vi "test_Local Chassis Number of Slots Property.vi"(8 "error in (no error)":errorcluster, 11 "TestCase in":refnum<class "Scan Engine Scripting API Custom Device Unit Tests.lvclass">) -> (0 "error out":errorcluster, 3 "TestCase out":refnum<class "Scan Engine Scripting API Custom Device Unit Tests.lvclass">)   [LabVIEW 2020, in "Scan Engine Scripting API Custom Device Unit Tests.lvclass"]
uses:
  Scan Engine Scripting API Custom Device Unit Tests.lvclass
  Shared/Type Defs/Main Settings.ctl
  Shared/Type Defs/Local Chassis Settings.ctl
  Scan Engine Scripting API Custom Device Unit Tests.lvclass/Scan Engine Scripting API Custom Device Unit Tests.ctl
  <vilib>/addons/_JKI Toolkits/VI Tester/TestCase.llb/TestCase.lvclass
  Scripting/Scan Engine Scripting.lvlib
  Shared/SEECD Shared.lvlib
  C:/Program Files (x86)/National Instruments/LabVIEW 2020/vi.lib/addons/_JKI Toolkits/VI Tester/TestCase.llb/TestCase.lvclass
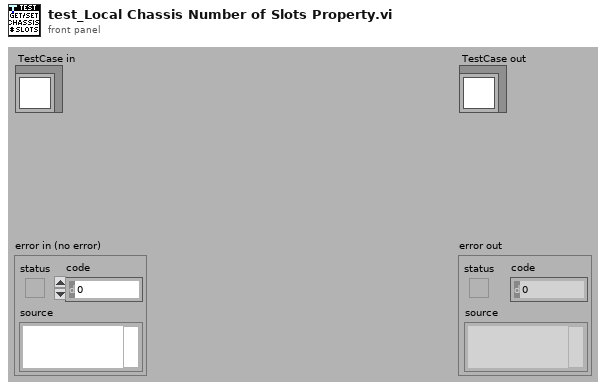
[diagram p1: front panel]
types:
  T1 = typedef "SEECD Shared.lvlib/Main Settings.ctl" = cluster{"sync to scan":bool, "scan engine decimation":u16, "delay after FPGA load (s)":u16}
  T2 = typedef "SEECD Shared.lvlib/Local Chassis Settings.ctl" = cluster{"name":string, "number of slots":i32}
  T3 = typedef "Custom Device API.lvlib/Custom Device Item Ref.ctl" = u64
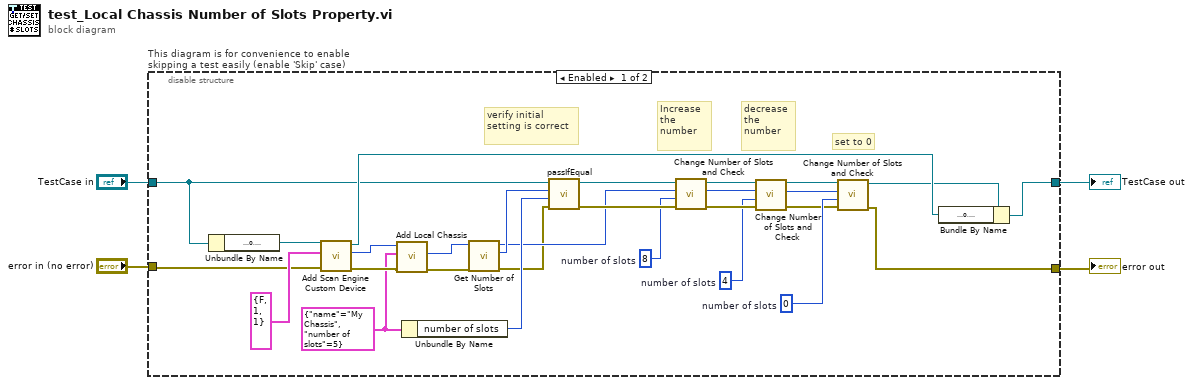
[diagram p0: block diagram]
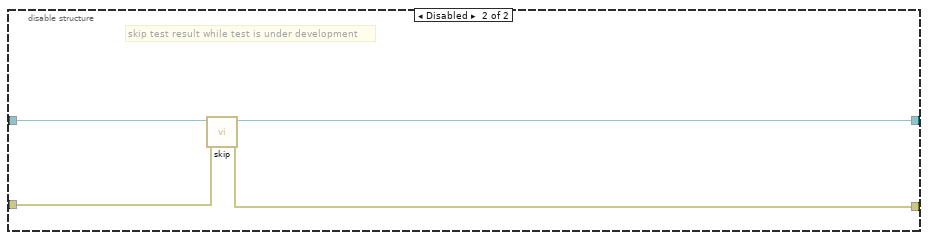
[diagram p2: hidden frame]
diagram:
  n1 = disable-structure "This diagram is for convenience to enable skipping a test easily (enable 'Skip' case)" shown="Enabled" {
    disable-tunnel: "TestCase in" -> [w22 w36]
    disable-tunnel: [w27 w34] -> w1
    disable-tunnel: [w9 w35] -> w3
    disable-tunnel: "error in (no error)" -> [w29 w33]
    frame Enabled {
      w14 = 0  # number of slots
      w15 = 4  # number of slots
      w18 = 8  # number of slots
      w26 = T2 {"name"="My Chassis", "number of slots"=5} ("settings")
      # "verify initial setting is correct"
      # "set to 0"
      # "decrease the number"
      # "Increase the number"
      n2 = Unbundle By Name(w22) -> ("target ref"=w28:refnum<k24>)
      n3 = call "Add Scan Engine Custom Device.vi"("error in"=w29, "settings"=T1 {"sync to scan"=FALSE, "scan engine decimation"=1, "delay after FPGA load (s)"=1}, "target in"=w28) -> ("error out"=w31:errorcluster, "scan engine custom device ref"=w30:T3, "target out"=w23:refnum<k24>)  [unwired: 6 in]
      n4 = call "Add Local Chassis.vi"("error in"=w31, "settings"=w26, "scan engine custom device ref in"=w30) -> ("error out"=w24:errorcluster, "local chassis ref"=w25:T3)  [unwired: 4 in, 3 out]
      n5 = Unbundle By Name(w26) -> ("number of slots"=w21:i32)
      n6 = call "Get Number of Slots.vi"("error in"=w24, "chassis ref in"=w25) -> ("error out"=w5:errorcluster, "number of slots"=w20:i32, "chassis ref out"=w6:T3)  [unwired: 7 in]
      n7 = call-dynamic "passIfEqual.vi"("error in (no error)"=w5, "y"=w21, "x"=w20, "TestCase in"=w22) -> ("error out"=w19:errorcluster, "TestCase out"=w8:refnum<class "Scan Engine Scripting API Custom Device Unit Tests.lvclass">)  [unwired: 6 in]
      n8 = call "Change Number of Slots and Check.vi"("error in"=w19, "number of slots"=w18, "chassis ref in"=w6, "test case in"=w8) -> ("error out"=w17:errorcluster, "chassis ref out"=w16:T3, "test case out"=w7:refnum<class "Scan Engine Scripting API Custom Device Unit Tests.lvclass">)  [unwired: 5 in]
      n9 = call "Change Number of Slots and Check.vi"("error in"=w17, "number of slots"=w15, "chassis ref in"=w16, "test case in"=w7) -> ("error out"=w11:errorcluster, "chassis ref out"=w12:T3, "test case out"=w13:refnum<class "Scan Engine Scripting API Custom Device Unit Tests.lvclass">)  [unwired: 5 in]
      n10 = call "Change Number of Slots and Check.vi"("error in"=w11, "number of slots"=w14, "chassis ref in"=w12, "test case in"=w13) -> ("error out"=w9:errorcluster, "test case out"=w10:refnum<class "Scan Engine Scripting API Custom Device Unit Tests.lvclass">)  [unwired: 5 in, 1 out]
      n11 = Bundle By Name(cluster=w10, "target ref"=w23) -> (w27:refnum<class "Scan Engine Scripting API Custom Device Unit Tests.lvclass">)
    }
    frame Disabled {
      # "skip test result while test is under development"
      n12 = call <vilib>:"skip.vi"("error in (no error)"=w33, "TestCase in"=w36) -> ("error out"=w35:errorcluster, "TestCase out"=w34:refnum<class "Scan Engine Scripting API Custom Device Unit Tests.lvclass">)  [unwired: 8 in]
    }
  }
  "error out" <- w3
  "TestCase out" <- w1
